vi "Find VI with Focus - Test Support - Setup.vi"(8 "error in (no error)":errorcluster) -> (0 "error out":errorcluster, 2 "VI Name":string, 3 "VI Renum":refnum<vi>)   [LabVIEW 2009]
doc: "This VI opens the front panel of a Test Support VI so it can be searched for it memory."
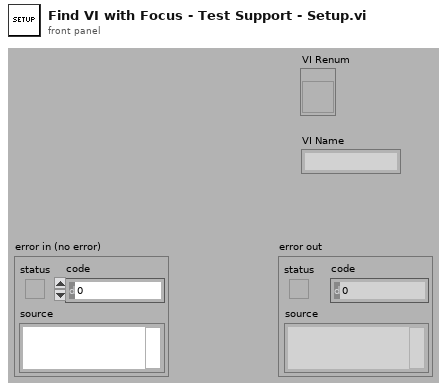
[diagram p1: front panel]
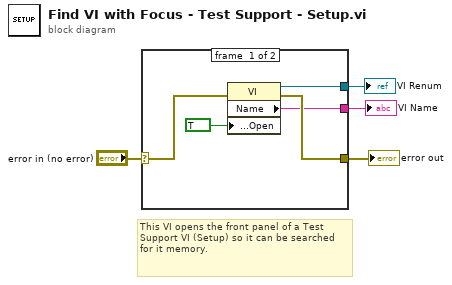
[diagram p0: block diagram]
diagram:
  # "This VI opens the front panel of a Test Support VI (Setup) so it can be searched for it memory."
  n1 = case shown="No Error" "error in (no error)" {
    selector: "error in (no error)" -> [w7 w10]
    tunnel: [w5 _] -> w4
    tunnel: [w9 _] -> w3
    tunnel: [w6 w10] -> w1
    frame #0 {
      n2 = property class="VI"(error in=w7, "Front Panel.Open"=TRUE ("Front Panel Window:Open")) -> (reference out=w9:refnum<vi>, error out=w6:errorcluster, "Name"=w5:string)  [unwired: 1 in]
    }
    frame #1 {
    }
  }
  "VI Name" <- w4
  "error out" <- w1
  "VI Renum" <- w3
